vi "send-loop.vi"(5 "set":bool[](array[boolean])=[TRUE, TRUE], 7 "loop":string[](array[string])=["60", "70"], 10 "case-in":bool, 11 "队列输入":refnum<queue>) -> (3 "dup Message Queue":refnum<queue>)   [LabVIEW 2015]
uses:
  <userlib>/QMH/Message Queue/Support/Message Cluster.ctl
  <userlib>/QMH/Message Queue/Support/Enqueue Message (Array).vi
  <userlib>/QMH/Message Queue/Message Queue.lvlib
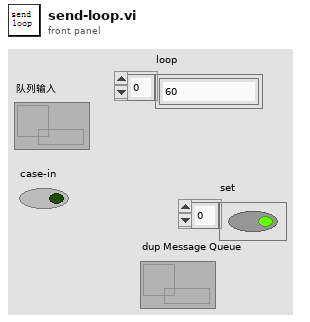
[diagram p1: front panel]
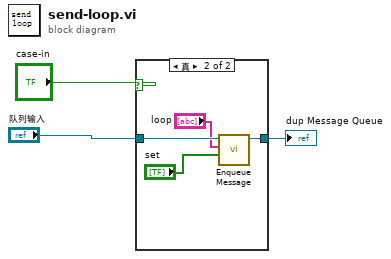
[diagram p0: block diagram]
diagram:
  n1 = case shown="真" "case-in" {
    tunnel: "队列输入" -> [w4 w8]
    tunnel: [w4 w6] -> w2
    frame False {
    }
    frame True {
      n2 = call-poly <userlib>:"Enqueue Message.vi"("Message Data Array"="set", "Message Array"="loop", "Message Queue"=w8) -> ("dup Message Queue"=w6:refnum<queue>)  [unwired: 7 in, 1 out]
    }
  }
  "dup Message Queue" <- w2
